vi "Plot_FFID_Calibs.vi"() -> ()   [LabVIEW 2014]
panel:
  out "Calib 2":cluster{dbl[], dbl[]}[](graph)
  out "Zero":cluster{dbl[], dbl[]}[](graph)
  out "Calib 1":cluster{dbl[], dbl[]}[](graph)
  in  "History (days)":i32=5 min=0
  out "Calib 3":cluster{dbl[], dbl[]}[](graph)
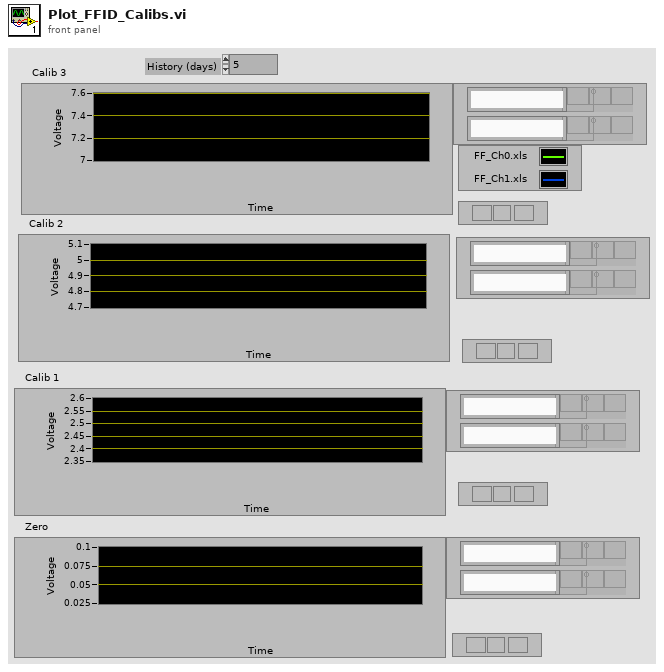
[diagram p1: front panel]
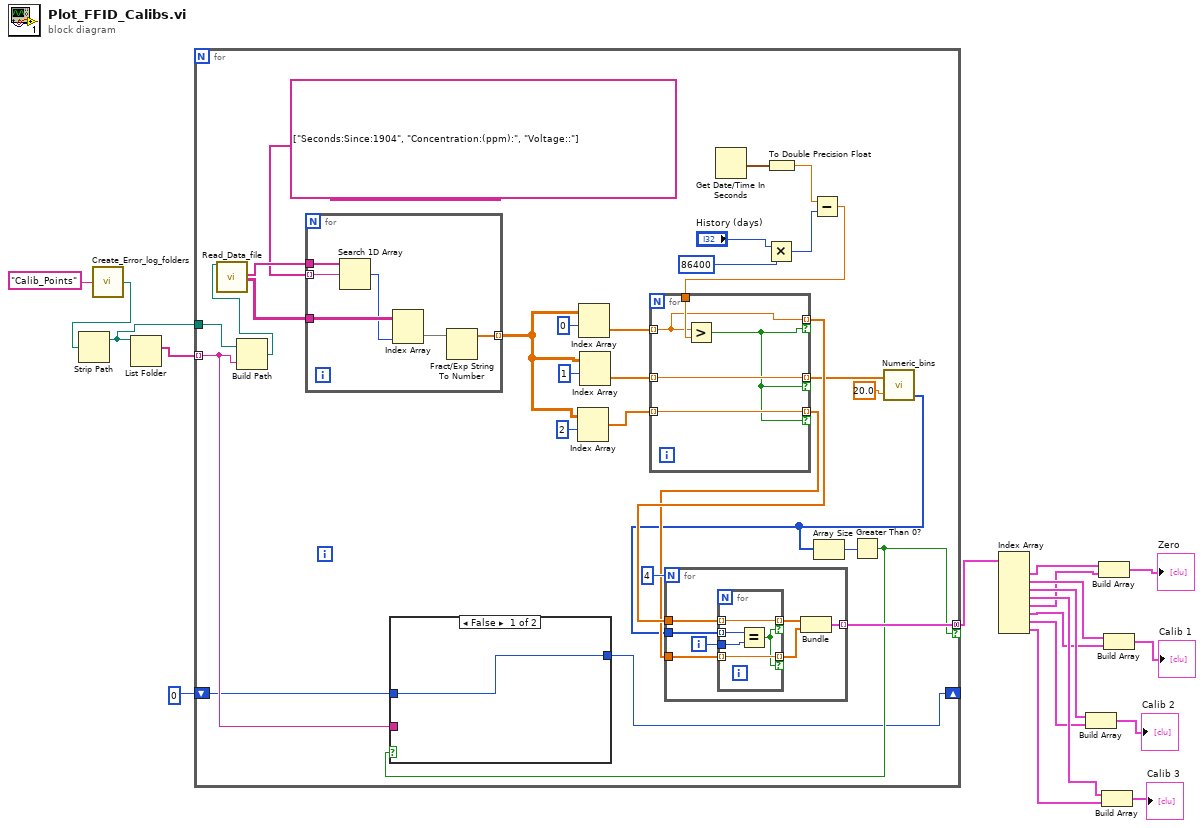
[diagram p0: block diagram]
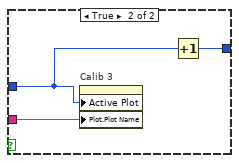
[diagram p2: hidden frame]
diagram:
  n1 = call "Create_Error_log_folders.vi"("Log Folder"="Calib_Points") -> ("Server copy Location"=w16:path)  [unwired: 2 in, 2 out]
  n2 = Strip Path(path=w16) -> (stripped path=w17:path)  [unwired: 1 out]
  n3 = List Folder(path=w17) -> (filenames=w11:string[])  [unwired: 3 in, 3 out]
  n4 = for {
    tunnel: w17 -> [w44]
    tunnel: w11 -> [w21] mode=indexing
    tunnel: [w25] -> w15 mode=concatenating if=w22
    shift-right: [w19] -> _
    shift-left: 0 -> [w20]
    n5 = Build Path(base path=w44, name or relative path=w21) -> (appended path=w43:path)
    n6 = call "Read_Data_file.vi"("Results file"=w43) -> ("Ch names Out"=w48:string[], "Channel Values Out"=w46:string[][])  [unwired: 9 in, 8 out]
    n7 = for {
      tunnel: w48 -> [w75]
      tunnel: string[] ["Seconds:Since:1904", "Concentration:(ppm):", "Voltage::"] ("Ch names Out") -> [w74] mode=indexing
      tunnel: w46 -> [w73]
      tunnel: [w70] -> w40 mode=indexing
      n8 = Search 1D Array(1D array=w75, element=w74) -> (index of element=w71:i32)  [unwired: 1 in]
      n9 = Index Array(array=w73, index (col)=w71) -> (element=w72:string[])  [unwired: 1 in]
      n10 = Fract/Exp String To Number(string=w72) -> (number=w70:dbl[])  [unwired: 3 in, 1 out]
    }
    n11 = Index Array(array=w40, index (row)=2) -> (element=w27:dbl[])  [unwired: 1 in]
    n12 = Index Array(array=w40, index (row)=0) -> (element=w31:dbl[])  [unwired: 1 in]
    n13 = Index Array(array=w40, index (row)=1) -> (element=w28:dbl[])  [unwired: 1 in]
    n14 = Get Date/Time In Seconds() -> (seconds since 1Jan1904=w37:timestamp)
    n15 = Multiply(x="History (days)", y=86400) -> (x*y=w33:i32)
    n16 = To Double Precision Float(number=w37) -> (double precision float=w34:dbl)
    n17 = Subtract(x=w34, y=w33) -> (x-y=w32:dbl)
    n18 = for {
      tunnel: w31 -> [w56] mode=indexing
      tunnel: w32 -> [w57]
      tunnel: [w56] -> w30 mode=indexing if=w53
      tunnel: [w55] -> w29 mode=indexing if=w53
      tunnel: w28 -> [w55] mode=indexing
      tunnel: [w54] -> w26 mode=indexing if=w53
      tunnel: w27 -> [w54] mode=indexing
      n19 = Greater?(x=w56, y=w57) -> (0:w53:bool)
    }
    n20 = call "Numeric_bins.vi"("Values"=w29, "Tolerance"=20.0) -> ("Bin Index"=w24:i32[])  [unwired: 2 out]
    n21 = for {
      N: 4 -> [_]
      tunnel: w24 -> [w64]
      tunnel: w30 -> [w61]
      tunnel: w26 -> [w60]
      tunnel: [w58] -> w25 mode=indexing
      i -> [w59]
      n22 = for {
        tunnel: w59 -> [w69]
        tunnel: w64 -> [w68] mode=indexing
        tunnel: [w67] -> w63 mode=indexing if=w65
        tunnel: w60 -> [w67] mode=indexing
        tunnel: [w66] -> w62 mode=indexing if=w65
        tunnel: w61 -> [w66] mode=indexing
        n23 = Equal?(x=w68, y=w69) -> (x = y?=w65:bool)
      }
      n24 = Bundle(w62, w63) -> (w58:cluster{dbl[], dbl[]})  [unwired: 1 in]
    }
    n25 = Array Size(array=w24) -> (size(s)=w23:i32)
    n26 = Greater Than 0?(x=w23) -> (x > 0?=w22:bool)
    n27 = case shown="False" w22 {
      tunnel: w21 -> [_ w52]
      tunnel: w20 -> [w49 w51]
      tunnel: [w49 w50] -> w19
      frame False {
      }
      frame True {
        n28 = property on="Calib 3" class="XYGraph (strict)"("Active Plot"=w51, "Plot.Plot Name"=w52) -> ()  [unwired: 2 in, 2 out]
        n29 = Increment(x=w51) -> (x+1=w50:i32)
      }
    }
  }
  n30 = Index Array(array=w15) -> (element #1=w14:cluster{dbl[], dbl[]}, element #2=w13:cluster{dbl[], dbl[]}, element #3=w7:cluster{dbl[], dbl[]}, element #4=w6:cluster{dbl[], dbl[]}, element #5=w5:cluster{dbl[], dbl[]}, element #6=w4:cluster{dbl[], dbl[]}, element #7=w3:cluster{dbl[], dbl[]}, element #8=w2:cluster{dbl[], dbl[]})  [unwired: 8 in]
  n31 = Build Array(w7, w3) -> (→"Calib 2":cluster{dbl[], dbl[]}[])
  n32 = Build Array(w14, w5) -> (→"Zero":cluster{dbl[], dbl[]}[])
  n33 = Build Array(w6, w2) -> (→"Calib 3":cluster{dbl[], dbl[]}[])
  n34 = Build Array(w13, w4) -> (→"Calib 1":cluster{dbl[], dbl[]}[])
